vi "HandleObservationSync.vi"(8 "error in (no error)":errorcluster, 11 "S4GUI in":refnum<class "S4GUI.lvclass">) -> (0 "error out":errorcluster, 3 "S4GUI out":refnum<class "S4GUI.lvclass">)   [LabVIEW 2018, in "S4GUI.lvclass"] (continued)
              n1024 = call-dynamic "Read State Machine.vi"("error in (no error)"=w2764, "Device in"=w2765) -> ("error out"=w2763:errorcluster, "State Machine.lvclass"=w2761:refnum<class "State Machine.lvclass">, "Device out"=w2767:refnum<class "Channel.lvclass">)  [unwired: 7 in]
              n1025 = call "Next State.vi"("error in (no error)"=w2763, "New_State"=50, "State Machine in"=w2761) -> ("error out"=w2755:errorcluster, "State Machine out"=w2754:refnum<class "State Machine.lvclass">)  [unwired: 7 in]
              n1026 = call-dynamic "Write State Machine.vi"("error in (no error)"=w2755, "State Machine.lvclass"=w2754, "Device in"=w2767) -> ("error out"=w2768:errorcluster, "Device out"=w2766:refnum<class "Channel.lvclass">)  [unwired: 7 in]
              n1027 = call-dynamic "Write Channel.vi"("error in (no error)"=w2768, "Channel.lvclass"=w2766, "Acquisition in"=w2758) -> ("error out"=w2760:errorcluster, "Acquisition out"=w2759:refnum<class "Acquisition.lvclass">)  [unwired: 7 in]
            }
          }
          n1028 = call-dynamic "Write AcquisitionC.vi"("error in (no error)"=w2679, "Acquisition.lvclass"=w2677, "S4ACS_GUI in"=w2678) -> ("error out"=w2673:errorcluster, "S4ACS_GUI out"=w2672:refnum<class "S4GUI.lvclass">)  [unwired: 7 in]
          n1029 = call-dynamic "Read AcquisitionD.vi"("error in (no error)"=w2673, "S4ACS_GUI in"=w2672) -> ("error out"=w2629:errorcluster, "Acquisition.lvclass"=w2631:refnum<class "Acquisition.lvclass">, "S4ACS_GUI out"=w2671:refnum<class "S4GUI.lvclass">)  [unwired: 7 in]
          n1030 = call-dynamic "Read enabled.vi"("error in (no error)"=w2629, "Server in"=w2631) -> ("error out"=w2628:errorcluster, "enabled"=w2624:bool, "Server out"=w2630:refnum<class "Acquisition.lvclass">)  [unwired: 7 in]
          n1031 = call "Read connection.vi"("error in (no error)"=w2628, "Server in"=w2630) -> ("error out"=w2660:errorcluster, "connection"=w2644:bool, "Server out"=w2661:refnum<class "Acquisition.lvclass">)  [unwired: 7 in]
          n1032 = And(x=w2644, y=w2624) -> (x .and. y?=w2646:bool)
          n1033 = case shown="True" w2646 {
            tunnel: w2660 -> [w2729 w2746]
            tunnel: [w2729 w2745] -> w2674
            tunnel: w2661 -> [w2730 w2736]
            tunnel: [w2730 w2734] -> w2670
            tunnel: [w2726 u32 0 ("New_State")] -> w2653
            tunnel: w2624 -> [w2725 _]
            frame False {
              n1034 = Select(t=u32 8, s=w2725, f=u32 0) -> (s? t:f=w2726:u32)
            }
            frame True {
              n1035 = call-dynamic "Read Channel.vi"("error in (no error)"=w2746, "Acquisition in"=w2736) -> ("error out"=w2741:errorcluster, "Channel.lvclass"=w2740:refnum<class "Channel.lvclass">, "Acquisition out"=w2735:refnum<class "Acquisition.lvclass">)  [unwired: 7 in]
              n1036 = call-dynamic "Read State Machine.vi"("error in (no error)"=w2741, "Device in"=w2740) -> ("error out"=w2742:errorcluster, "State Machine.lvclass"=w2744:refnum<class "State Machine.lvclass">, "Device out"=w2738:refnum<class "Channel.lvclass">)  [unwired: 7 in]
              n1037 = call "Next State.vi"("error in (no error)"=w2742, "New_State"=50, "State Machine in"=w2744) -> ("error out"=w2732:errorcluster, "State Machine out"=w2733:refnum<class "State Machine.lvclass">)  [unwired: 7 in]
              n1038 = call-dynamic "Write State Machine.vi"("error in (no error)"=w2732, "State Machine.lvclass"=w2733, "Device in"=w2738) -> ("error out"=w2737:errorcluster, "Device out"=w2739:refnum<class "Channel.lvclass">)  [unwired: 7 in]
              n1039 = call-dynamic "Write Channel.vi"("error in (no error)"=w2737, "Channel.lvclass"=w2739, "Acquisition in"=w2735) -> ("error out"=w2745:errorcluster, "Acquisition out"=w2734:refnum<class "Acquisition.lvclass">)  [unwired: 7 in]
            }
          }
          n1040 = call-dynamic "Write AcquisitionD.vi"("error in (no error)"=w2674, "Acquisition.lvclass"=w2670, "S4ACS_GUI in"=w2671) -> ("error out"=w2669:errorcluster, "S4ACS_GUI out"=w2668:refnum<class "S4GUI.lvclass">)  [unwired: 7 in]
          n1041 = Compound Arithmetic op=ADD(w2656, w2655, w2654, w2653) -> (w2657:u32)
          n1042 = case shown="0, Default" w2657 {
            tunnel: w2652 -> [w2694 _ _ _ _ _ _ _ _ _ _ _ _ _ _ _]
            tunnel: [w2693 u32 1 ("Obs_state") u32 1 ("Obs_state") u32 1 ("Obs_state") u32 1 ("Obs_state") u32 1 ("Obs_state") u32 1 ("Obs_state") u32 1 ("Obs_state") u32 1 ("Obs_state") u32 1 ("Obs_state") u32 1 ("Obs_state") u32 1 ("Obs_state") u32 1 ("Obs_state") u32 1 ("Obs_state") u32 1 ("Obs_state") u32 1 ("Obs_state")] -> w2658
            tunnel: ["" ("Error Msg") "ERROR: Lost channel 1 connection... - HandleObservationSync.vi state 308" ("Error Msg") "ERROR: Lost channel 2 connection...- HandleObservationSync.vi state 308" ("Error Msg") "ERROR: Lost channels 1 and 2 connection...- HandleObservationSync.vi state 308" ("Error Msg") "ERROR: Lost channel 3 connection...- HandleObservationSync.vi state 308" ("Error Msg") "ERROR: Lost channels 1 and  3 connection...- HandleObservationSync.vi state 308" ("Error Msg") "ERROR:  Lost channels 2 and  3 connection...- HandleObservationSync.vi state 308" ("Error Msg") "ERROR:  Lost channels 1, 2 and  3 connection...- HandleObservationSync.vi state 308" ("Error Msg") "ERROR: Lost channel 4 connection...- HandleObservationSync.vi state 308" ("Error Msg") "ERROR:  Lost channels 1 and 4 connection...- HandleObservationSync.vi state 308" ("Error Msg") "ERROR:  Lost channels 2 and 4 connection...- HandleObservationSync.vi state 308" ("Error Msg") "ERROR: Lost channels 1, 2 and 4 connection...- HandleObservationSync.vi state 308" ("Error Msg") "ERROR: Lost channels 3 and 4 connection...- HandleObservationSync.vi state 308" ("Error Msg") "ERROR: Lost channels 1, 3 and 4 connection...- HandleObservationSync.vi state 308" ("Error Msg") "ERROR: Lost channels 2, 3 and 4 connection...- HandleObservationSync.vi state 308" ("Error Msg") "ERROR: Lost channels 1, 2, 3 and 4 connection...- HandleObservationSync.vi state 308" ("Error Msg")] -> w2659
            frame 0, Default {
              n1043 = Tick Count (ms)() -> (millisecond timer value=w2691:u32)
              n1044 = Increment(x=w2694) -> (x+1=w2693:u32)
              n1045 = local write "time1"(w2691) -> ()
            }
            frame 1 {
            }
            frame 2 {
            }
            frame 3 {
            }
            frame 4 {
            }
            frame 5 {
            }
            frame 6 {
            }
            frame 7 {
            }
            frame 8 {
            }
            frame 9 {
            }
            frame 10 {
            }
            frame 11 {
            }
            frame 12 {
            }
            frame 13 {
            }
            frame 14 {
            }
            frame 15 {
            }
          }
          n1046 = Bundle By Name(cluster=w2668, "Obs_state"=w2658, "Error Msg"=w2659) -> (w2685:refnum<class "S4GUI.lvclass">)
        }
        frame 309 {
          # "Se wait_expose=T, não envia\no EXPOSE do estado 310\n(1o EXPOSE já foi enviado).\n\nNeste caso, vai para:\n* 310 se houver mais \n   de 1 posição da lamina ou para \n* 327 se houver apenas 1 posição\n   da lâmina"
          # "T: mode EXPOSE\nF: mode FIRE"
          n1047 = Unbundle By Name(w2819) -> ("seqAtual"=w2818:u32)
          n1048 = call-dynamic "Read AcquisitionA.vi"("error in (no error)"=w2879, "S4ACS_GUI in"=w2819) -> ("error out"=w2859:errorcluster, "Acquisition.lvclass"=w2860:refnum<class "Acquisition.lvclass">, "S4ACS_GUI out"=w2881:refnum<class "S4GUI.lvclass">)  [unwired: 7 in]
          n1049 = call "Read connection.vi"("error in (no error)"=w2859, "Server in"=w2860) -> ("error out"=w2861:errorcluster, "connection"=w2863:bool, "Server out"=w2862:refnum<class "Acquisition.lvclass">)  [unwired: 7 in]
          n1050 = case shown="True" w2863 {
            tunnel: [w3032 w3056] -> w2882
            tunnel: [w3031 w3055] -> w2880
            tunnel: w2862 -> [w3032 w3048]
            tunnel: w2861 -> [w3031 w3047]
            tunnel: [TRUE w3046] -> w2842
            tunnel: [FALSE w3040] -> w2838
            tunnel: [TRUE w3034] -> w2823
            tunnel: w2818 -> [_ w3033]
            frame False {
            }
            frame True {
              n1051 = call-dynamic "Read Channel.vi"("error in (no error)"=w3047, "Acquisition in"=w3048) -> ("error out"=w3037:errorcluster, "Channel.lvclass"=w3039:refnum<class "Channel.lvclass">, "Acquisition out"=w3057:refnum<class "Acquisition.lvclass">)  [unwired: 7 in]
              n1052 = call-dynamic "Read SequesDone.vi"("error in (no error)"=w3037, "Channel in"=w3039) -> ("error out"=w3036:errorcluster, "SequesDoneRaw"=w3035:u32, "Channel out"=w3038:refnum<class "Channel.lvclass">)  [unwired: 6 in, 1 out]
              n1053 = Equal?(x=w3035, y=w3033) -> (x = y?=w3034:bool)
              n1054 = call-dynamic "Read wait_expose.vi"("error in (no error)"=w3036, "Channel in"=w3038) -> ("error out"=w3041:errorcluster, "wait_expose"=w3040:bool, "Channel out"=w3042:refnum<class "Channel.lvclass">)  [unwired: 7 in]
              n1055 = call-dynamic "Read State Machine.vi"("error in (no error)"=w3041, "Device in"=w3042) -> ("error out"=w3049:errorcluster, "State Machine.lvclass"=w3051:refnum<class "State Machine.lvclass">, "Device out"=w3053:refnum<class "Channel.lvclass">)  [unwired: 7 in]
              n1056 = call-dynamic "Read State.vi"("error in (no error)"=w3049, "State Machine in"=w3051) -> ("error out"=w3043:errorcluster, "State"=w3045:i32, "State Machine out"=w3050:refnum<class "State Machine.lvclass">)  [unwired: 7 in]
              n1057 = Greater?(x=w3045, y=53) -> (0:w3046:bool)
              n1058 = call-dynamic "Write State Machine.vi"("error in (no error)"=w3043, "State Machine.lvclass"=w3050, "Device in"=w3053) -> ("error out"=w3052:errorcluster, "Device out"=w3054:refnum<class "Channel.lvclass">)  [unwired: 7 in]
              n1059 = call-dynamic "Write Channel.vi"("error in (no error)"=w3052, "Channel.lvclass"=w3054, "Acquisition in"=w3057) -> ("error out"=w3055:errorcluster, "Acquisition out"=w3056:refnum<class "Acquisition.lvclass">)  [unwired: 7 in]
            }
          }
          n1060 = call-dynamic "Write AcquisitionA.vi"("error in (no error)"=w2880, "Acquisition.lvclass"=w2882, "S4ACS_GUI in"=w2881) -> ("error out"=w2876:errorcluster, "S4ACS_GUI out"=w2877:refnum<class "S4GUI.lvclass">)  [unwired: 7 in]
          n1061 = call "Read AcquisitionB.vi"("error in (no error)"=w2876, "S4ACS_GUI in"=w2877) -> ("error out"=w2856:errorcluster, "Acquisition.lvclass"=w2858:refnum<class "Acquisition.lvclass">, "S4ACS_GUI out"=w2874:refnum<class "S4GUI.lvclass">)  [unwired: 7 in]
          n1062 = call "Read connection.vi"("error in (no error)"=w2856, "Server in"=w2858) -> ("error out"=w2855:errorcluster, "connection"=w2854:bool, "Server out"=w2857:refnum<class "Acquisition.lvclass">)  [unwired: 7 in]
          n1063 = case shown="True" w2854 {
            tunnel: w2857 -> [w3002 w3027]
            tunnel: w2855 -> [w3001 w3026]
            tunnel: [w3002 w3024] -> w2875
            tunnel: [w3001 w3023] -> w2873
            tunnel: [TRUE w3014] -> w2841
            tunnel: [FALSE ("expose") w3010] -> w2837
            tunnel: [TRUE w3004] -> w2825
            tunnel: w2818 -> [_ w3003]
            frame False {
            }
            frame True {
              n1064 = call-dynamic "Read Channel.vi"("error in (no error)"=w3026, "Acquisition in"=w3027) -> ("error out"=w3006:errorcluster, "Channel.lvclass"=w3009:refnum<class "Channel.lvclass">, "Acquisition out"=w3025:refnum<class "Acquisition.lvclass">)  [unwired: 7 in]
              n1065 = call-dynamic "Read SequesDone.vi"("error in (no error)"=w3006, "Channel in"=w3009) -> ("error out"=w3005:errorcluster, "SequesDoneRaw"=w3007:u32, "Channel out"=w3008:refnum<class "Channel.lvclass">)  [unwired: 6 in, 1 out]
              n1066 = Equal?(x=w3007, y=w3003) -> (x = y?=w3004:bool)
              n1067 = call-dynamic "Read wait_expose.vi"("error in (no error)"=w3005, "Channel in"=w3008) -> ("error out"=w3011:errorcluster, "wait_expose"=w3010:bool, "Channel out"=w3012:refnum<class "Channel.lvclass">)  [unwired: 7 in]
              n1068 = call-dynamic "Read State Machine.vi"("error in (no error)"=w3011, "Device in"=w3012) -> ("error out"=w3017:errorcluster, "State Machine.lvclass"=w3019:refnum<class "State Machine.lvclass">, "Device out"=w3021:refnum<class "Channel.lvclass">)  [unwired: 7 in]
              n1069 = call-dynamic "Read State.vi"("error in (no error)"=w3017, "State Machine in"=w3019) -> ("error out"=w3016:errorcluster, "State"=w3013:i32, "State Machine out"=w3018:refnum<class "State Machine.lvclass">)  [unwired: 7 in]
              n1070 = Greater?(x=w3013, y=53) -> (0:w3014:bool)
              n1071 = call-dynamic "Write State Machine.vi"("error in (no error)"=w3016, "State Machine.lvclass"=w3018, "Device in"=w3021) -> ("error out"=w3020:errorcluster, "Device out"=w3022:refnum<class "Channel.lvclass">)  [unwired: 7 in]
              n1072 = call-dynamic "Write Channel.vi"("error in (no error)"=w3020, "Channel.lvclass"=w3022, "Acquisition in"=w3025) -> ("error out"=w3023:errorcluster, "Acquisition out"=w3024:refnum<class "Acquisition.lvclass">)  [unwired: 7 in]
            }
          }
          n1073 = call "Write AcquisitionB.vi"("error in (no error)"=w2873, "Acquisition.lvclass"=w2875, "S4ACS_GUI in"=w2874) -> ("error out"=w2869:errorcluster, "S4ACS_GUI out"=w2868:refnum<class "S4GUI.lvclass">)  [unwired: 7 in]
          n1074 = call-dynamic "Read AcquisitionC.vi"("error in (no error)"=w2869, "S4ACS_GUI in"=w2868) -> ("error out"=w2851:errorcluster, "Acquisition.lvclass"=w2853:refnum<class "Acquisition.lvclass">, "S4ACS_GUI out"=w2871:refnum<class "S4GUI.lvclass">)  [unwired: 7 in]
          n1075 = call "Read connection.vi"("error in (no error)"=w2851, "Server in"=w2853) -> ("error out"=w2850:errorcluster, "connection"=w2849:bool, "Server out"=w2852:refnum<class "Acquisition.lvclass">)  [unwired: 7 in]
          n1076 = case shown="True" w2849 {
            tunnel: [w2971 w2992] -> w2872
            tunnel: [w2972 w2991] -> w2870
            tunnel: w2852 -> [w2972 w2987]
            tunnel: w2850 -> [w2971 w2986]
            tunnel: [TRUE w2983] -> w2840
            tunnel: [FALSE ("expose") w2980] -> w2836
            tunnel: [TRUE w2974] -> w2824
            tunnel: w2818 -> [_ w2973]
            frame False {
            }
            frame True {
              n1077 = call-dynamic "Read Channel.vi"("error in (no error)"=w2986, "Acquisition in"=w2987) -> ("error out"=w2979:errorcluster, "Channel.lvclass"=w2978:refnum<class "Channel.lvclass">, "Acquisition out"=w2990:refnum<class "Acquisition.lvclass">)  [unwired: 7 in]
              n1078 = call-dynamic "Read SequesDone.vi"("error in (no error)"=w2979, "Channel in"=w2978) -> ("error out"=w2975:errorcluster, "SequesDoneRaw"=w2976:u32, "Channel out"=w2977:refnum<class "Channel.lvclass">)  [unwired: 6 in, 1 out]
              n1079 = Equal?(x=w2976, y=w2973) -> (x = y?=w2974:bool)
              n1080 = call-dynamic "Read wait_expose.vi"("error in (no error)"=w2975, "Channel in"=w2977) -> ("error out"=w2981:errorcluster, "wait_expose"=w2980:bool, "Channel out"=w2982:refnum<class "Channel.lvclass">)  [unwired: 7 in]
              n1081 = call-dynamic "Read State Machine.vi"("error in (no error)"=w2981, "Device in"=w2982) -> ("error out"=w2988:errorcluster, "State Machine.lvclass"=w2996:refnum<class "State Machine.lvclass">, "Device out"=w2994:refnum<class "Channel.lvclass">)  [unwired: 7 in]
              n1082 = call-dynamic "Read State.vi"("error in (no error)"=w2988, "State Machine in"=w2996) -> ("error out"=w2989:errorcluster, "State"=w2984:i32, "State Machine out"=w2997:refnum<class "State Machine.lvclass">)  [unwired: 7 in]
              n1083 = Greater?(x=w2984, y=53) -> (0:w2983:bool)
              n1084 = call-dynamic "Write State Machine.vi"("error in (no error)"=w2989, "State Machine.lvclass"=w2997, "Device in"=w2994) -> ("error out"=w2995:errorcluster, "Device out"=w2993:refnum<class "Channel.lvclass">)  [unwired: 7 in]
              n1085 = call-dynamic "Write Channel.vi"("error in (no error)"=w2995, "Channel.lvclass"=w2993, "Acquisition in"=w2990) -> ("error out"=w2992:errorcluster, "Acquisition out"=w2991:refnum<class "Acquisition.lvclass">)  [unwired: 7 in]
            }
          }
          n1086 = call-dynamic "Write AcquisitionC.vi"("error in (no error)"=w2872, "Acquisition.lvclass"=w2870, "S4ACS_GUI in"=w2871) -> ("error out"=w2848:errorcluster, "S4ACS_GUI out"=w2864:refnum<class "S4GUI.lvclass">)  [unwired: 7 in]
          n1087 = call-dynamic "Read AcquisitionD.vi"("error in (no error)"=w2848, "S4ACS_GUI in"=w2864) -> ("error out"=w2844:errorcluster, "Acquisition.lvclass"=w2847:refnum<class "Acquisition.lvclass">, "S4ACS_GUI out"=w2866:refnum<class "S4GUI.lvclass">)  [unwired: 7 in]
          n1088 = call "Read connection.vi"("error in (no error)"=w2844, "Server in"=w2847) -> ("error out"=w2845:errorcluster, "connection"=w2843:bool, "Server out"=w2846:refnum<class "Acquisition.lvclass">)  [unwired: 7 in]
          n1089 = case shown="True" w2843 {
            tunnel: [w2942 w2966] -> w2867
            tunnel: [w2941 w2965] -> w2865
            tunnel: [TRUE w2954] -> w2839
            tunnel: w2846 -> [w2942 w2957]
            tunnel: w2845 -> [w2941 w2956]
            tunnel: [FALSE ("expose") w2950] -> w2835
            tunnel: [TRUE w2944] -> w2826
            tunnel: w2818 -> [_ w2943]
            frame False {
            }
            frame True {
              n1090 = call-dynamic "Read Channel.vi"("error in (no error)"=w2956, "Acquisition in"=w2957) -> ("error out"=w2948:errorcluster, "Channel.lvclass"=w2949:refnum<class "Channel.lvclass">, "Acquisition out"=w2967:refnum<class "Acquisition.lvclass">)  [unwired: 7 in]
              n1091 = call-dynamic "Read SequesDone.vi"("error in (no error)"=w2948, "Channel in"=w2949) -> ("error out"=w2946:errorcluster, "SequesDoneRaw"=w2947:u32, "Channel out"=w2945:refnum<class "Channel.lvclass">)  [unwired: 6 in, 1 out]
              n1092 = Equal?(x=w2947, y=w2943) -> (x = y?=w2944:bool)
              n1093 = call-dynamic "Read wait_expose.vi"("error in (no error)"=w2946, "Channel in"=w2945) -> ("error out"=w2951:errorcluster, "wait_expose"=w2950:bool, "Channel out"=w2952:refnum<class "Channel.lvclass">)  [unwired: 7 in]
              n1094 = call-dynamic "Read State Machine.vi"("error in (no error)"=w2951, "Device in"=w2952) -> ("error out"=w2959:errorcluster, "State Machine.lvclass"=w2961:refnum<class "State Machine.lvclass">, "Device out"=w2963:refnum<class "Channel.lvclass">)  [unwired: 7 in]
              n1095 = call-dynamic "Read State.vi"("error in (no error)"=w2959, "State Machine in"=w2961) -> ("error out"=w2958:errorcluster, "State"=w2953:i32, "State Machine out"=w2960:refnum<class "State Machine.lvclass">)  [unwired: 7 in]
              n1096 = Greater?(x=w2953, y=53) -> (0:w2954:bool)
              n1097 = call-dynamic "Write State Machine.vi"("error in (no error)"=w2958, "State Machine.lvclass"=w2960, "Device in"=w2963) -> ("error out"=w2962:errorcluster, "Device out"=w2964:refnum<class "Channel.lvclass">)  [unwired: 7 in]
              n1098 = call-dynamic "Write Channel.vi"("error in (no error)"=w2962, "Channel.lvclass"=w2964, "Acquisition in"=w2967) -> ("error out"=w2965:errorcluster, "Acquisition out"=w2966:refnum<class "Acquisition.lvclass">)  [unwired: 7 in]
            }
          }
          n1099 = call-dynamic "Write AcquisitionD.vi"("error in (no error)"=w2865, "Acquisition.lvclass"=w2867, "S4ACS_GUI in"=w2866) -> ("error out"=w2817:errorcluster, "S4ACS_GUI out"=w2815:refnum<class "S4GUI.lvclass">)  [unwired: 7 in]
          n1100 = Compound Arithmetic op=OR(w2838, w2837, w2836, w2835) -> (w2828:bool)
          n1101 = Compound Arithmetic op=AND(w2823, w2825, w2824, w2826) -> (w2821:bool)
          n1102 = Compound Arithmetic op=AND(w2842, w2841, w2840, w2839) -> (w2822:bool)
          n1103 = disable-structure shown="Enabled" {
            disable-tunnel: w2822 -> [w2885 w2886]
            disable-tunnel: w2821 -> [w2884 _]
            disable-tunnel: [w2883 w2886] -> w2820
            frame Disabled {
              # "Espera todos os canais chegarem ao estado ACTIVE\n(estados 54 e 55 de Channel:Run.vi)\n   OU\nTodos os canais incrementarem o Seqs_done. (OV 20240821)"
              n1104 = Or(x=w2885, y=w2884) -> (x .or. y?=w2883:bool)
            }
            frame Enabled {
              # "OV20241108:\nEspera APENAS o ACTIVE."
            }
          }
          n1105 = call-dynamic "VerifErrors.vi"("error in (no error)"=w2817, "S4GUI in"=w2815) -> ("error out"=w2816:errorcluster, "Error value"=w2813:u32, "S4GUI out"=w2814:refnum<class "S4GUI.lvclass">)  [unwired: 7 in]
          n1106 = call-dynamic "VerifWavePlate.vi"("error in (no error)"=w2816, "S4GUI in"=w2814) -> ("error out"=w2832:errorcluster, "One Position"=w2834:bool, "S4GUI out"=w2833:refnum<class "S4GUI.lvclass">)  [unwired: 7 in]
          n1107 = case shown="False" w2834 {
            tunnel: w2833 -> [w2919 w2936]
            tunnel: [u32 312 ("t") u32 328 ("t")] -> w2830
            tunnel: [w2919 w2922] -> w2829
            tunnel: w2832 -> [w2917 w2921]
            tunnel: [w2917 w2920] -> w2831
            frame False {
            }
            frame True {
              # "Recarrega SEQ, antes de desviar\n para tratamento de fotometria."
              n1108 = call "Read Instrument.lvclass.vi"("error in (no error)"=w2921, "S4ACS_GUI in"=w2936) -> ("error out"=w2931:errorcluster, "Instrument.lvclass"=w2935:refnum<class "Instrument.lvclass">, "S4ACS_GUI out"=w2934:refnum<class "S4GUI.lvclass">)  [unwired: 7 in]
              n1109 = call "Read WPROT.vi"("error in (no error)"=w2931, "Instrument in"=w2935) -> ("error out"=w2924:errorcluster, "Opt_Selector.lvclass"=w2927:refnum<class "Opt_Selector.lvclass">, "Instrument out"=w2932:refnum<class "Instrument.lvclass">)  [unwired: 7 in]
              n1110 = call-dynamic "Read sequencia_ant.vi"("error in (no error)"=w2924, "Opt_Selector in"=w2927) -> ("error out"=w2929:errorcluster, "sequencia_ant"=w2928:u16, "Opt_Selector out"=w2926:refnum<class "Opt_Selector.lvclass">)  [unwired: 7 in]
              n1111 = call-dynamic "Write sequencia.vi"("error in (no error)"=w2929, "sequencia"=w2928, "Opt_Selector in"=w2926) -> ("error out"=w2923:errorcluster, "Opt_Selector out"=w2925:refnum<class "Opt_Selector.lvclass">)  [unwired: 7 in]
              n1112 = call "Write WPROT.vi"("error in (no error)"=w2923, "Opt_Selector.lvclass"=w2925, "Instrument in"=w2932) -> ("error out"=w2930:errorcluster, "Instrument out"=w2933:refnum<class "Instrument.lvclass">)  [unwired: 7 in]
              n1113 = call "Write Instrument.lvclass.vi"("error in (no error)"=w2930, "Instrument.lvclass"=w2933, "S4ACS_GUI in"=w2934) -> ("error out"=w2920:errorcluster, "S4ACS_GUI out"=w2922:refnum<class "S4GUI.lvclass">)  [unwired: 7 in]
            }
          }
          n1114 = case shown="False" w2820 {
            tunnel: w2829 -> [w2889 w2916]
            tunnel: [w2895 w2915] -> w2827
            tunnel: w2830 -> [_ w2913]
            tunnel: w2813 -> [w2887 _]
            frame False {
              # "Aguardando iniciar exposição por 5s"
              n1115 = Tick Count (ms)() -> (millisecond timer value=w2894:u32)
              n1116 = local read "time1"() -> (w2888:u32)
              n1117 = Subtract(x=w2894, y=w2888) -> (x-y=w2891:u32)
              n1118 = To Double Precision Float(number=w2891) -> (double precision float=w2893:dbl)
              n1119 = Less?(x=5000.0 ("y"), y=w2893) -> (x < y?=w2892:bool)
              n1120 = case shown="False" w2892 {
                tunnel: w2889 -> [w2897 w2911]
                tunnel: [w2896 w2910] -> w2895
                tunnel: w2887 -> [w2898 _]
                frame False {
                  n1121 = case shown="1..15" w2898 {
                    selector: w2898 -> [_ w2906]
                    tunnel: [w2899 w2901] -> w2896
                    tunnel: w2897 -> [w2899 w2907]
                    frame 0, Default {
                    }
                    frame 1..15 {
                      n1122 = Number To Decimal String(number=w2906) -> (decimal integer string=w2903:string)  [unwired: 1 in]
                      n1123 = Concatenate Strings("CHANNEL ERROR <", w2903, ">: Error flag TRUE - see ACS panel.  HandleObservationSync.vi - state 309.") -> (w2905:string)
                      n1124 = Bundle By Name(cluster=w2907, "Obs_state"=u32 1, "Error Msg"=w2905) -> (w2901:refnum<class "S4GUI.lvclass">)
                    }
                  }
                }
                frame True {
                  n1125 = Bundle By Name(cluster=w2911, "Obs_state"=u32 1, "Error Msg"="ERROR: Acquisition Timeout. HandleObservationSync.vi - state 309.") -> (w2910:refnum<class "S4GUI.lvclass">)
                }
              }
            }
            frame True {
              # "Iniciou aquisição..."
              n1126 = Tick Count (ms)() -> (millisecond timer value=→"time308":u32)
              n1127 = Tick Count (ms)() -> (millisecond timer value=w2914:u32)
              n1128 = Bundle By Name(cluster=w2916, "Obs_state"=w2913) -> (w2915:refnum<class "S4GUI.lvclass">)
              n1129 = local write "time307"(w2914) -> ()
              n1130 = local write "time1"(w2914) -> ()
            }
          }
          n1131 = Bundle By Name(cluster=w2827, "mode EXPOSE"=w2828) -> (w2878:refnum<class "S4GUI.lvclass">)
        }
        frame 312 {
          # "Verifcando avanço de SEQUENCIA:"
          # "T=canais receberam STOP"
          # "T= Todos os canais ativos na mesma sequencia;\nF= Canais com sequencia diferente"
          # "Todos os SEQ_DONE \nsão iguais a SeqAtual?\nSe sim, avança lâmina."
          # "Exemplo:\nSET #CYCLES 3\nSET #SEQ 4\ntotal de sequencias: 3 x 4 = 12\n\nseq.        CYCLES_DONE           SEQS_DONE\n1a.                     0                                 0\n2a.                     0                                 1 \n3a.                     0                                 2 \n4a.                     0                                 3 \n                          1                                 4\n5a.                     1                                 0 \n6a.                     1                                 1 \n7a.                     1                                 2 \n8a.                     1                                 3 \n                          2                                 4\n9a.                     2                                 0 \n10a.                   2                                 1 \n11a.                   2                                 2 \n12a.                   2                                 3 \n\nfim                    3                                 4"
          n1132 = Unbundle By Name(w3083) -> ("seqAtual"=w3080:u32)
          n1133 = call-dynamic "Read AcquisitionA.vi"("error in (no error)"=w3117, "S4ACS_GUI in"=w3083) -> ("error out"=w3098:errorcluster, "Acquisition.lvclass"=w3099:refnum<class "Acquisition.lvclass">, "S4ACS_GUI out"=w3119:refnum<class "S4GUI.lvclass">)  [unwired: 7 in]
          n1134 = call-dynamic "Read enabled.vi"("error in (no error)"=w3098, "Server in"=w3099) -> ("error out"=w3097:errorcluster, "enabled"=w3072:bool, "Server out"=w3096:refnum<class "Acquisition.lvclass">)  [unwired: 7 in]
          n1135 = case shown="True" w3072 {
            tunnel: w3097 -> [w3268 w3284]
            tunnel: [w3269 w3282] -> w3120
            tunnel: [w3268 w3281] -> w3118
            tunnel: [u32 0 ("SequesDone") w3270] -> w3077
            tunnel: w3096 -> [w3269 w3280]
            tunnel: w3080 -> [_ w3279]
            tunnel: [TRUE w3278] -> w3082
            tunnel: [FALSE ("stopping") w3271] -> w3065
            frame False {
            }
            frame True {
              # "SEQS_DONE = 0,1,2,...,n,0,1,..."
              n1136 = call-dynamic "Read Channel.vi"("error in (no error)"=w3284, "Acquisition in"=w3280) -> ("error out"=w3276:errorcluster, "Channel.lvclass"=w3277:refnum<class "Channel.lvclass">, "Acquisition out"=w3283:refnum<class "Acquisition.lvclass">)  [unwired: 7 in]
              n1137 = call-dynamic "Read SequesDone.vi"("error in (no error)"=w3276, "Channel in"=w3277) -> ("error out"=w3274:errorcluster, "SequesDoneRaw"=w3270:u32, "Channel out"=w3275:refnum<class "Channel.lvclass">)  [unwired: 6 in, 1 out]
              n1138 = Equal?(x=w3270, y=w3279) -> (x = y?=w3278:bool)
              n1139 = call-dynamic "Read stopping.vi"("error in (no error)"=w3274, "Channel in"=w3275) -> ("error out"=w3273:errorcluster, "stopping"=w3271:bool, "Channel out"=w3272:refnum<class "Channel.lvclass">)  [unwired: 7 in]
              n1140 = call-dynamic "Write Channel.vi"("error in (no error)"=w3273, "Channel.lvclass"=w3272, "Acquisition in"=w3283) -> ("error out"=w3281:errorcluster, "Acquisition out"=w3282:refnum<class "Acquisition.lvclass">)  [unwired: 7 in]
            }
          }
          n1141 = call-dynamic "Write AcquisitionA.vi"("error in (no error)"=w3118, "Acquisition.lvclass"=w3120, "S4ACS_GUI in"=w3119) -> ("error out"=w3115:errorcluster, "S4ACS_GUI out"=w3114:refnum<class "S4GUI.lvclass">)  [unwired: 7 in]
          n1142 = call "Read AcquisitionB.vi"("error in (no error)"=w3115, "S4ACS_GUI in"=w3114) -> ("error out"=w3092:errorcluster, "Acquisition.lvclass"=w3095:refnum<class "Acquisition.lvclass">, "S4ACS_GUI out"=w3116:refnum<class "S4GUI.lvclass">)  [unwired: 7 in]
          n1143 = call-dynamic "Read enabled.vi"("error in (no error)"=w3092, "Server in"=w3095) -> ("error out"=w3093:errorcluster, "enabled"=w3071:bool, "Server out"=w3094:refnum<class "Acquisition.lvclass">)  [unwired: 7 in]
          n1144 = case shown="True" w3071 {
            tunnel: w3093 -> [w3248 w3264]
            tunnel: w3094 -> [w3249 w3263]
            tunnel: [u32 0 ("SequesDone") w3250] -> w3074
            tunnel: [w3248 w3262] -> w3113
            tunnel: [w3249 w3261] -> w3112
            tunnel: w3080 -> [_ w3258]
            tunnel: [TRUE w3257] -> w3081
            tunnel: [FALSE ("stopping") w3251] -> w3064
            frame False {
            }
            frame True {
              n1145 = call-dynamic "Read Channel.vi"("error in (no error)"=w3264, "Acquisition in"=w3263) -> ("error out"=w3255:errorcluster, "Channel.lvclass"=w3256:refnum<class "Channel.lvclass">, "Acquisition out"=w3259:refnum<class "Acquisition.lvclass">)  [unwired: 7 in]
              n1146 = call-dynamic "Read SequesDone.vi"("error in (no error)"=w3255, "Channel in"=w3256) -> ("error out"=w3253:errorcluster, "SequesDoneRaw"=w3250:u32, "Channel out"=w3260:refnum<class "Channel.lvclass">)  [unwired: 6 in, 1 out]
              n1147 = Equal?(x=w3250, y=w3258) -> (x = y?=w3257:bool)
              n1148 = call-dynamic "Read stopping.vi"("error in (no error)"=w3253, "Channel in"=w3260) -> ("error out"=w3252:errorcluster, "stopping"=w3251:bool, "Channel out"=w3254:refnum<class "Channel.lvclass">)  [unwired: 7 in]
              n1149 = call-dynamic "Write Channel.vi"("error in (no error)"=w3252, "Channel.lvclass"=w3254, "Acquisition in"=w3259) -> ("error out"=w3262:errorcluster, "Acquisition out"=w3261:refnum<class "Acquisition.lvclass">)  [unwired: 7 in]
            }
          }
          n1150 = call "Write AcquisitionB.vi"("error in (no error)"=w3113, "Acquisition.lvclass"=w3112, "S4ACS_GUI in"=w3116) -> ("error out"=w3105:errorcluster, "S4ACS_GUI out"=w3104:refnum<class "S4GUI.lvclass">)  [unwired: 7 in]
          n1151 = call-dynamic "Read AcquisitionC.vi"("error in (no error)"=w3105, "S4ACS_GUI in"=w3104) -> ("error out"=w3089:errorcluster, "Acquisition.lvclass"=w3091:refnum<class "Acquisition.lvclass">, "S4ACS_GUI out"=w3107:refnum<class "S4GUI.lvclass">)  [unwired: 7 in]
          n1152 = call-dynamic "Read enabled.vi"("error in (no error)"=w3089, "Server in"=w3091) -> ("error out"=w3088:errorcluster, "enabled"=w3070:bool, "Server out"=w3090:refnum<class "Acquisition.lvclass">)  [unwired: 7 in]
          n1153 = case shown="True" w3070 {
            tunnel: [w3228 w3244] -> w3108
            tunnel: [w3229 w3243] -> w3106
            tunnel: w3088 -> [w3228 w3240]
            tunnel: w3090 -> [w3229 w3241]
            tunnel: [u32 0 ("SequesDone") w3230] -> w3073
            tunnel: w3080 -> [_ w3239]
            tunnel: [TRUE w3238] -> w3079
            tunnel: [FALSE ("stopping") w3231] -> w3063
            frame False {
            }
            frame True {
              n1154 = call-dynamic "Read Channel.vi"("error in (no error)"=w3240, "Acquisition in"=w3241) -> ("error out"=w3235:errorcluster, "Channel.lvclass"=w3236:refnum<class "Channel.lvclass">, "Acquisition out"=w3242:refnum<class "Acquisition.lvclass">)  [unwired: 7 in]
              n1155 = call-dynamic "Read SequesDone.vi"("error in (no error)"=w3235, "Channel in"=w3236) -> ("error out"=w3233:errorcluster, "SequesDoneRaw"=w3230:u32, "Channel out"=w3237:refnum<class "Channel.lvclass">)  [unwired: 6 in, 1 out]
              n1156 = Equal?(x=w3230, y=w3239) -> (x = y?=w3238:bool)
              n1157 = call-dynamic "Read stopping.vi"("error in (no error)"=w3233, "Channel in"=w3237) -> ("error out"=w3232:errorcluster, "stopping"=w3231:bool, "Channel out"=w3234:refnum<class "Channel.lvclass">)  [unwired: 7 in]
              n1158 = call-dynamic "Write Channel.vi"("error in (no error)"=w3232, "Channel.lvclass"=w3234, "Acquisition in"=w3242) -> ("error out"=w3244:errorcluster, "Acquisition out"=w3243:refnum<class "Acquisition.lvclass">)  [unwired: 7 in]
            }
          }
          n1159 = call-dynamic "Write AcquisitionC.vi"("error in (no error)"=w3108, "Acquisition.lvclass"=w3106, "S4ACS_GUI in"=w3107) -> ("error out"=w3102:errorcluster, "S4ACS_GUI out"=w3103:refnum<class "S4GUI.lvclass">)  [unwired: 7 in]
          n1160 = call-dynamic "Read AcquisitionD.vi"("error in (no error)"=w3102, "S4ACS_GUI in"=w3103) -> ("error out"=w3085:errorcluster, "Acquisition.lvclass"=w3087:refnum<class "Acquisition.lvclass">, "S4ACS_GUI out"=w3109:refnum<class "S4GUI.lvclass">)  [unwired: 7 in]
          n1161 = call-dynamic "Read enabled.vi"("error in (no error)"=w3085, "Server in"=w3087) -> ("error out"=w3084:errorcluster, "enabled"=w3069:bool, "Server out"=w3086:refnum<class "Acquisition.lvclass">)  [unwired: 7 in]
          n1162 = Build Array(w3072, w3071, w3070, w3069) -> (w3068:bool[])
          n1163 = case shown="True" w3069 {
            tunnel: [w3209 w3224] -> w3111
            tunnel: [w3208 w3223] -> w3110
            tunnel: w3086 -> [w3209 w3222]
            tunnel: w3084 -> [w3208 w3221]
            tunnel: [u32 0 ("SequesDone") w3210] -> w3076
            tunnel: w3080 -> [_ w3219]
            tunnel: [TRUE w3218] -> w3078
            tunnel: [FALSE ("stopping") w3211] -> w3062
            frame False {
            }
            frame True {
              n1164 = call-dynamic "Read Channel.vi"("error in (no error)"=w3221, "Acquisition in"=w3222) -> ("error out"=w3215:errorcluster, "Channel.lvclass"=w3216:refnum<class "Channel.lvclass">, "Acquisition out"=w3220:refnum<class "Acquisition.lvclass">)  [unwired: 7 in]
              n1165 = call-dynamic "Read SequesDone.vi"("error in (no error)"=w3215, "Channel in"=w3216) -> ("error out"=w3213:errorcluster, "SequesDoneRaw"=w3210:u32, "Channel out"=w3217:refnum<class "Channel.lvclass">)  [unwired: 6 in, 1 out]
              n1166 = Equal?(x=w3210, y=w3219) -> (x = y?=w3218:bool)
              n1167 = call-dynamic "Read stopping.vi"("error in (no error)"=w3213, "Channel in"=w3217) -> ("error out"=w3212:errorcluster, "stopping"=w3211:bool, "Channel out"=w3214:refnum<class "Channel.lvclass">)  [unwired: 7 in]
              n1168 = call-dynamic "Write Channel.vi"("error in (no error)"=w3212, "Channel.lvclass"=w3214, "Acquisition in"=w3220) -> ("error out"=w3223:errorcluster, "Acquisition out"=w3224:refnum<class "Acquisition.lvclass">)  [unwired: 7 in]
            }
          }
          n1169 = Boolean Array To Number(Boolean array=w3068) -> (number=w3066:u32)
          n1170 = Compound Arithmetic op=AND(w3082, w3081, w3079, w3078) -> (w3067:bool)
          n1171 = Compound Arithmetic op=OR(w3065, w3064, w3063, w3062) -> (w3061:bool)
          n1172 = case shown="11" w3066 {
            tunnel: w3077 -> [w3128 _ w3140 _ w3149 _ w3155 w3161 _ w3167 w3170 _]
            tunnel: w3076 -> [w3127 w3131 w3136 w3143 w3144 w3152 w3154 _ _ _ _ _]
            tunnel: w3074 -> [w3126 w3129 _ _ w3148 w3150 _ w3160 w3164 _ w3169 _]
            tunnel: w3073 -> [w3125 w3130 w3135 w3141 _ _ _ w3159 w3163 w3166 _ _]
            tunnel: [w3121 w3132 w3137 w3142 w3145 w3151 w3153 w3156 w3162 w3165 w3168 TRUE] -> _
            frame 15 {
              # "A,B,C,D ativos"
              n1173 = Equal?(x=w3128, y=w3126) -> (x = y?=w3124:bool)
              n1174 = Equal?(x=w3125, y=w3127) -> (x = y?=w3122:bool)
              n1175 = Equal?(x=w3126, y=w3125) -> (x = y?=w3123:bool)
              n1176 = Compound Arithmetic op=AND(w3124, w3123, w3122) -> (w3121:bool)
            }
            frame 14 {
              # "B,C e,D ativos"
              n1177 = Equal?(x=w3129, y=w3130) -> (x = y?=w3134:bool)
              n1178 = Equal?(x=w3130, y=w3131) -> (x = y?=w3133:bool)
              n1179 = Compound Arithmetic op=AND(w3134, w3133) -> (w3132:bool)
            }
            frame 13 {
              # "A,C e,D ativos"
              n1180 = Equal?(x=w3140, y=w3135) -> (x = y?=w3139:bool)
              n1181 = Equal?(x=w3135, y=w3136) -> (x = y?=w3138:bool)
              n1182 = Compound Arithmetic op=AND(w3139, w3138) -> (w3137:bool)
            }
            frame 12 {
              # "Só C e D ativos"
              n1183 = Equal?(x=w3141, y=w3143) -> (x = y?=w3142:bool)
            }
            frame 11 {
              # "A,B e,D ativos"
              n1184 = Equal?(x=w3149, y=w3148) -> (x = y?=w3147:bool)
              n1185 = Equal?(x=w3148, y=w3144) -> (x = y?=w3146:bool)
              n1186 = Compound Arithmetic op=AND(w3147, w3146) -> (w3145:bool)
            }
            frame 10 {
              # "Só B e D ativos"
              n1187 = Equal?(x=w3150, y=w3152) -> (x = y?=w3151:bool)
            }
            frame 9 {
              # "Só A e D ativos"
              n1188 = Equal?(x=w3155, y=w3154) -> (x = y?=w3153:bool)
            }
            frame 7 {
              # "A,B,C ativos"
              n1189 = Equal?(x=w3161, y=w3160) -> (x = y?=w3158:bool)
              n1190 = Equal?(x=w3160, y=w3159) -> (x = y?=w3157:bool)
              n1191 = Compound Arithmetic op=AND(w3158, w3157) -> (w3156:bool)
            }
            frame 6 {
              # "Só B e C ativos"
              n1192 = Equal?(x=w3164, y=w3163) -> (x = y?=w3162:bool)
            }
            frame 5 {
              # "Só A e C ativos"
              n1193 = Equal?(x=w3167, y=w3166) -> (x = y?=w3165:bool)
            }
            frame 3 {
              # "só A e B ativos"
              n1194 = Equal?(x=w3170, y=w3169) -> (x = y?=w3168:bool)
            }
            frame 0..2, 4, 8, Default {
              # "nenhum ou só 1  \ncanal ativo."
            }
          }
          n1195 = call-dynamic "Write AcquisitionD.vi"("error in (no error)"=w3110, "Acquisition.lvclass"=w3111, "S4ACS_GUI in"=w3109) -> ("error out"=w3100:errorcluster, "S4ACS_GUI out"=w3101:refnum<class "S4GUI.lvclass">)  [unwired: 7 in]
          n1196 = And(x=w3067, y=TRUE) -> (x .and. y?=w3075:bool)
          n1197 = case shown="True" w3075 {
            tunnel: w3101 -> [w3173 w3202]
            tunnel: [w3172 w3201] -> w3060
            tunnel: w3067 -> [w3174 _]
            tunnel: w3061 -> [_ w3200]
            tunnel: w3059 -> [_ w3195]
            frame False {
              n1198 = case shown="True" w3174 {
                tunnel: w3173 -> [w3181 w3194]
                tunnel: [w3185 w3193] -> w3172
                frame False {
                  # "Esperando todos os canais habilitados mudarem de sequesDone.\nE verificando a maior duracao de cubo entre os canais."
                  n1199 = local read "time307"() -> (w3184:u32)
                  n1200 = Tick Count (ms)() -> (millisecond timer value=w3183:u32)
                  n1201 = Subtract(x=w3183, y=w3184) -> (x-y=w3178:u32)
                  n1202 = call-dynamic "GetGreatestCube.vi"("S4GUI in"=w3181) -> ("S4GUI out"=w3180:refnum<class "S4GUI.lvclass">, "greatest (ms)"=w3176:dbl)  [unwired: 8 in, 1 out]
                  n1203 = To Double Precision Float(number=w3178) -> (double precision float=w3182:dbl)
                  n1204 = Add(x=1000.0 ("y"), y=w3176) -> (x+y=w3175:dbl)
                  n1205 = Less?(x=w3175, y=w3182) -> (x < y?=w3179:bool)
                  n1206 = case shown="True" w3179 {
                    tunnel: w3180 -> [w3186 w3190]
                    tunnel: [w3186 w3189] -> w3185
                    frame False {
                    }
                    frame True {
                      n1207 = Bundle By Name(cluster=w3190, "Obs_state"=u32 1, "Error Msg"="ERROR: Acquisition Timeout - HandleObservationSync.vi - state 312.") -> (w3189:refnum<class "S4GUI.lvclass">)
                    }
                  }
                }
                frame True {
                  # "Nunca entra aqui!!"
                  n1208 = Bundle By Name(cluster=w3194, "Obs_state"=u32 1, "Error Msg"="ERROR: Sequence_done not equal in all active channels.") -> (w3193:refnum<class "S4GUI.lvclass">)
                }
              }
            }
            frame True {
              # "STOP?"
              n1209 = local read "time308"() -> (w3198:u32)
              n1210 = Tick Count (ms)() -> (millisecond timer value=w3199:u32)
              n1211 = Subtract(x=w3199, y=w3198) -> (x-y=→"delay Acq":u32)
              n1212 = case shown="False" w3200 {
                tunnel: w3195 -> [_ _]
                tunnel: [u32 303 u32 0] -> w3196
                frame False {
                }
                frame True {
                }
              }
              n1213 = Bundle By Name(cluster=w3202, "Obs_state"=w3196) -> (w3201:refnum<class "S4GUI.lvclass">)
            }
          }
        }
        frame 314 {
          n1214 = Unbundle By Name(w3288) -> ("cyclesDone"=w3286:u32)
          n1215 = Increment(x=w3286) -> (x+1=w3285:u32)
          n1216 = Bundle By Name(cluster=w3288, "cyclesDone"=w3285) -> (w3287:refnum<class "S4GUI.lvclass">)
          n1217 = Unbundle By Name(w3287) -> ("TotalCiclos"=w3295:u32, "cyclesDone"=w3294:u32)
          n1218 = Subtract(x=w3295, y=w3294) -> (x-y=w3293:u32)
          n1219 = Greater Than 0?(x=w3293) -> (x > 0?=w3292:bool)
          n1220 = Select(t=u32 303, s=w3292, f=u32 0) -> (s? t:f=w3291:u32)
          n1221 = Bundle By Name(cluster=w3287, "Obs_state"=w3291) -> (w3296:refnum<class "S4GUI.lvclass">)
        }
        frame 321 {
          n1222 = call-dynamic "Read AcquisitionA.vi"("error in (no error)"=w3360, "S4ACS_GUI in"=w3361) -> ("error out"=w3315:errorcluster, "Acquisition.lvclass"=w3316:refnum<class "Acquisition.lvclass">, "S4ACS_GUI out"=w3363:refnum<class "S4GUI.lvclass">)  [unwired: 7 in]
          n1223 = call-dynamic "Read enabled.vi"("error in (no error)"=w3315, "Server in"=w3316) -> ("error out"=w3314:errorcluster, "enabled"=w3301:bool, "Server out"=w3317:refnum<class "Acquisition.lvclass">)  [unwired: 7 in]
          n1224 = call "Read connection.vi"("error in (no error)"=w3314, "Server in"=w3317) -> ("error out"=w3340:errorcluster, "connection"=w3324:bool, "Server out"=w3341:refnum<class "Acquisition.lvclass">)  [unwired: 7 in]
          n1225 = And(x=w3324, y=w3301) -> (x .and. y?=w3325:bool)
          n1226 = case shown="True" w3325 {
            tunnel: w3341 -> [w3478 w3497]
            tunnel: w3340 -> [w3477 w3496]
            tunnel: [w3478 w3494] -> w3364
            tunnel: [w3477 w3493] -> w3362
            tunnel: [w3474 u32 0 ("New_State")] -> w3330
            tunnel: w3301 -> [w3473 _]
            frame False {
              n1227 = Select(t=u32 1, s=w3473, f=u32 0) -> (s? t:f=w3474:u32)
            }
            frame True {
              n1228 = call-dynamic "Read Channel.vi"("error in (no error)"=w3496, "Acquisition in"=w3497) -> ("error out"=w3480:errorcluster, "Channel.lvclass"=w3483:refnum<class "Channel.lvclass">, "Acquisition out"=w3495:refnum<class "Acquisition.lvclass">)  [unwired: 7 in]
              n1229 = call-dynamic "Write wait_expose.vi"("error in (no error)"=w3480, "wait_expose"=TRUE, "Channel in"=w3483) -> ("error out"=w3479:errorcluster, "Channel out"=w3482:refnum<class "Channel.lvclass">)  [unwired: 7 in]
              n1230 = call-dynamic "Read State Machine.vi"("error in (no error)"=w3479, "Device in"=w3482) -> ("error out"=w3490:errorcluster, "State Machine.lvclass"=w3492:refnum<class "State Machine.lvclass">, "Device out"=w3488:refnum<class "Channel.lvclass">)  [unwired: 7 in]
              n1231 = call "Next State.vi"("error in (no error)"=w3490, "New_State"=40, "State Machine in"=w3492) -> ("error out"=w3485:errorcluster, "State Machine out"=w3486:refnum<class "State Machine.lvclass">)  [unwired: 7 in]
              n1232 = call-dynamic "Write State Machine.vi"("error in (no error)"=w3485, "State Machine.lvclass"=w3486, "Device in"=w3488) -> ("error out"=w3487:errorcluster, "Device out"=w3489:refnum<class "Channel.lvclass">)  [unwired: 7 in]
              n1233 = call-dynamic "Write Channel.vi"("error in (no error)"=w3487, "Channel.lvclass"=w3489, "Acquisition in"=w3495) -> ("error out"=w3493:errorcluster, "Acquisition out"=w3494:refnum<class "Acquisition.lvclass">)  [unwired: 7 in]
            }
          }
          n1234 = call-dynamic "Write AcquisitionA.vi"("error in (no error)"=w3362, "Acquisition.lvclass"=w3364, "S4ACS_GUI in"=w3363) -> ("error out"=w3357:errorcluster, "S4ACS_GUI out"=w3358:refnum<class "S4GUI.lvclass">)  [unwired: 7 in]
          n1235 = call "Read AcquisitionB.vi"("error in (no error)"=w3357, "S4ACS_GUI in"=w3358) -> ("error out"=w3311:errorcluster, "Acquisition.lvclass"=w3313:refnum<class "Acquisition.lvclass">, "S4ACS_GUI out"=w3355:refnum<class "S4GUI.lvclass">)  [unwired: 7 in]
          n1236 = call-dynamic "Read enabled.vi"("error in (no error)"=w3311, "Server in"=w3313) -> ("error out"=w3310:errorcluster, "enabled"=w3300:bool, "Server out"=w3312:refnum<class "Acquisition.lvclass">)  [unwired: 7 in]
          n1237 = call "Read connection.vi"("error in (no error)"=w3310, "Server in"=w3312) -> ("error out"=w3338:errorcluster, "connection"=w3322:bool, "Server out"=w3339:refnum<class "Acquisition.lvclass">)  [unwired: 7 in]
          n1238 = And(x=w3322, y=w3300) -> (x .and. y?=w3323:bool)
          n1239 = case shown="True" w3323 {
            tunnel: w3339 -> [w3453 w3472]
            tunnel: w3338 -> [w3452 w3471]
            tunnel: [w3453 w3469] -> w3356
            tunnel: [w3452 w3468] -> w3354
            tunnel: [w3449 u32 0 ("New_State")] -> w3329
            tunnel: w3300 -> [w3448 _]
            frame False {
              n1240 = Select(t=u32 2, s=w3448, f=u32 0) -> (s? t:f=w3449:u32)
            }
            frame True {
              n1241 = call-dynamic "Read Channel.vi"("error in (no error)"=w3471, "Acquisition in"=w3472) -> ("error out"=w3455:errorcluster, "Channel.lvclass"=w3457:refnum<class "Channel.lvclass">, "Acquisition out"=w3470:refnum<class "Acquisition.lvclass">)  [unwired: 7 in]
              n1242 = call-dynamic "Write wait_expose.vi"("error in (no error)"=w3455, "wait_expose"=TRUE, "Channel in"=w3457) -> ("error out"=w3454:errorcluster, "Channel out"=w3456:refnum<class "Channel.lvclass">)  [unwired: 7 in]
              n1243 = call-dynamic "Read State Machine.vi"("error in (no error)"=w3454, "Device in"=w3456) -> ("error out"=w3465:errorcluster, "State Machine.lvclass"=w3467:refnum<class "State Machine.lvclass">, "Device out"=w3463:refnum<class "Channel.lvclass">)  [unwired: 7 in]
              n1244 = call "Next State.vi"("error in (no error)"=w3465, "New_State"=40, "State Machine in"=w3467) -> ("error out"=w3460:errorcluster, "State Machine out"=w3461:refnum<class "State Machine.lvclass">)  [unwired: 7 in]
              n1245 = call-dynamic "Write State Machine.vi"("error in (no error)"=w3460, "State Machine.lvclass"=w3461, "Device in"=w3463) -> ("error out"=w3462:errorcluster, "Device out"=w3464:refnum<class "Channel.lvclass">)  [unwired: 7 in]
              n1246 = call-dynamic "Write Channel.vi"("error in (no error)"=w3462, "Channel.lvclass"=w3464, "Acquisition in"=w3470) -> ("error out"=w3468:errorcluster, "Acquisition out"=w3469:refnum<class "Acquisition.lvclass">)  [unwired: 7 in]
            }
          }
          n1247 = call "Write AcquisitionB.vi"("error in (no error)"=w3354, "Acquisition.lvclass"=w3356, "S4ACS_GUI in"=w3355) -> ("error out"=w3350:errorcluster, "S4ACS_GUI out"=w3349:refnum<class "S4GUI.lvclass">)  [unwired: 7 in]
          n1248 = call-dynamic "Read AcquisitionC.vi"("error in (no error)"=w3350, "S4ACS_GUI in"=w3349) -> ("error out"=w3307:errorcluster, "Acquisition.lvclass"=w3309:refnum<class "Acquisition.lvclass">, "S4ACS_GUI out"=w3352:refnum<class "S4GUI.lvclass">)  [unwired: 7 in]
          n1249 = call-dynamic "Read enabled.vi"("error in (no error)"=w3307, "Server in"=w3309) -> ("error out"=w3306:errorcluster, "enabled"=w3299:bool, "Server out"=w3308:refnum<class "Acquisition.lvclass">)  [unwired: 7 in]
          n1250 = call "Read connection.vi"("error in (no error)"=w3306, "Server in"=w3308) -> ("error out"=w3336:errorcluster, "connection"=w3319:bool, "Server out"=w3337:refnum<class "Acquisition.lvclass">)  [unwired: 7 in]
          n1251 = And(x=w3319, y=w3299) -> (x .and. y?=w3321:bool)
          n1252 = case shown="True" w3321 {
            tunnel: [w3427 w3441] -> w3353
            tunnel: [w3428 w3440] -> w3351
            tunnel: w3337 -> [w3428 w3438]
            tunnel: w3336 -> [w3427 w3437]
            tunnel: [w3424 u32 0 ("New_State")] -> w3328
            tunnel: w3299 -> [w3423 _]
            frame False {
              n1253 = Select(t=u32 4, s=w3423, f=u32 0) -> (s? t:f=w3424:u32)
            }
            frame True {
              n1254 = call-dynamic "Read Channel.vi"("error in (no error)"=w3437, "Acquisition in"=w3438) -> ("error out"=w3430:errorcluster, "Channel.lvclass"=w3432:refnum<class "Channel.lvclass">, "Acquisition out"=w3439:refnum<class "Acquisition.lvclass">)  [unwired: 7 in]
              n1255 = call-dynamic "Write wait_expose.vi"("error in (no error)"=w3430, "wait_expose"=TRUE, "Channel in"=w3432) -> ("error out"=w3429:errorcluster, "Channel out"=w3431:refnum<class "Channel.lvclass">)  [unwired: 7 in]
              n1256 = call-dynamic "Read State Machine.vi"("error in (no error)"=w3429, "Device in"=w3431) -> ("error out"=w3444:errorcluster, "State Machine.lvclass"=w3442:refnum<class "State Machine.lvclass">, "Device out"=w3446:refnum<class "Channel.lvclass">)  [unwired: 7 in]
              n1257 = call "Next State.vi"("error in (no error)"=w3444, "New_State"=40, "State Machine in"=w3442) -> ("error out"=w3436:errorcluster, "State Machine out"=w3435:refnum<class "State Machine.lvclass">)  [unwired: 7 in]
              n1258 = call-dynamic "Write State Machine.vi"("error in (no error)"=w3436, "State Machine.lvclass"=w3435, "Device in"=w3446) -> ("error out"=w3447:errorcluster, "Device out"=w3445:refnum<class "Channel.lvclass">)  [unwired: 7 in]
              n1259 = call-dynamic "Write Channel.vi"("error in (no error)"=w3447, "Channel.lvclass"=w3445, "Acquisition in"=w3439) -> ("error out"=w3441:errorcluster, "Acquisition out"=w3440:refnum<class "Acquisition.lvclass">)  [unwired: 7 in]
            }
          }
          n1260 = call-dynamic "Write AcquisitionC.vi"("error in (no error)"=w3353, "Acquisition.lvclass"=w3351, "S4ACS_GUI in"=w3352) -> ("error out"=w3347:errorcluster, "S4ACS_GUI out"=w3346:refnum<class "S4GUI.lvclass">)  [unwired: 7 in]
          n1261 = call-dynamic "Read AcquisitionD.vi"("error in (no error)"=w3347, "S4ACS_GUI in"=w3346) -> ("error out"=w3303:errorcluster, "Acquisition.lvclass"=w3305:refnum<class "Acquisition.lvclass">, "S4ACS_GUI out"=w3345:refnum<class "S4GUI.lvclass">)  [unwired: 7 in]
          n1262 = call-dynamic "Read enabled.vi"("error in (no error)"=w3303, "Server in"=w3305) -> ("error out"=w3302:errorcluster, "enabled"=w3298:bool, "Server out"=w3304:refnum<class "Acquisition.lvclass">)  [unwired: 7 in]
          n1263 = call "Read connection.vi"("error in (no error)"=w3302, "Server in"=w3304) -> ("error out"=w3334:errorcluster, "connection"=w3318:bool, "Server out"=w3335:refnum<class "Acquisition.lvclass">)  [unwired: 7 in]
          n1264 = And(x=w3318, y=w3298) -> (x .and. y?=w3320:bool)
          n1265 = case shown="True" w3320 {
            tunnel: w3334 -> [w3402 w3422]
            tunnel: [w3402 w3421] -> w3348
            tunnel: w3335 -> [w3403 w3414]
            tunnel: [w3403 w3412] -> w3344
            tunnel: [w3399 u32 0 ("New_State")] -> w3327
            tunnel: w3298 -> [w3398 _]
            frame False {
              n1266 = Select(t=u32 8, s=w3398, f=u32 0) -> (s? t:f=w3399:u32)
            }
            frame True {
              n1267 = call-dynamic "Read Channel.vi"("error in (no error)"=w3422, "Acquisition in"=w3414) -> ("error out"=w3404:errorcluster, "Channel.lvclass"=w3407:refnum<class "Channel.lvclass">, "Acquisition out"=w3413:refnum<class "Acquisition.lvclass">)  [unwired: 7 in]
              n1268 = call-dynamic "Write wait_expose.vi"("error in (no error)"=w3404, "wait_expose"=TRUE, "Channel in"=w3407) -> ("error out"=w3405:errorcluster, "Channel out"=w3406:refnum<class "Channel.lvclass">)  [unwired: 7 in]
              n1269 = call-dynamic "Read State Machine.vi"("error in (no error)"=w3405, "Device in"=w3406) -> ("error out"=w3418:errorcluster, "State Machine.lvclass"=w3420:refnum<class "State Machine.lvclass">, "Device out"=w3416:refnum<class "Channel.lvclass">)  [unwired: 7 in]
              n1270 = call "Next State.vi"("error in (no error)"=w3418, "New_State"=40, "State Machine in"=w3420) -> ("error out"=w3410:errorcluster, "State Machine out"=w3411:refnum<class "State Machine.lvclass">)  [unwired: 7 in]
              n1271 = call-dynamic "Write State Machine.vi"("error in (no error)"=w3410, "State Machine.lvclass"=w3411, "Device in"=w3416) -> ("error out"=w3415:errorcluster, "Device out"=w3417:refnum<class "Channel.lvclass">)  [unwired: 7 in]
              n1272 = call-dynamic "Write Channel.vi"("error in (no error)"=w3415, "Channel.lvclass"=w3417, "Acquisition in"=w3413) -> ("error out"=w3421:errorcluster, "Acquisition out"=w3412:refnum<class "Acquisition.lvclass">)  [unwired: 7 in]
            }
          }
          n1273 = call-dynamic "Write AcquisitionD.vi"("error in (no error)"=w3348, "Acquisition.lvclass"=w3344, "S4ACS_GUI in"=w3345) -> ("error out"=w3343:errorcluster, "S4ACS_GUI out"=w3342:refnum<class "S4GUI.lvclass">)  [unwired: 7 in]
          n1274 = Compound Arithmetic op=ADD(w3330, w3329, w3328, w3327) -> (w3331:u32)
          n1275 = case shown="0, Default" w3331 {
            tunnel: w3326 -> [w3367 _ _ _ _ _ _ _ _ _ _ _ _ _ _ _]
            tunnel: [w3366 u32 1 ("Obs_state") u32 1 ("Obs_state") u32 1 ("Obs_state") u32 1 ("Obs_state") u32 1 ("Obs_state") u32 1 ("Obs_state") u32 1 ("Obs_state") u32 1 ("Obs_state") u32 1 ("Obs_state") u32 1 ("Obs_state") u32 1 ("Obs_state") u32 1 ("Obs_state") u32 1 ("Obs_state") u32 1 ("Obs_state") u32 1 ("Obs_state")] -> w3332
            tunnel: ["" ("Error Msg") "ERROR: Lost channel 1 connection... - HandleObservationSync.vi state 321" ("Error Msg") "ERROR: Lost channel 2 connection...- HandleObservationSync.vi state 321" ("Error Msg") "ERROR: Lost channels 1 and 2 connection...- HandleObservationSync.vi state 321" ("Error Msg") "ERROR: Lost channel 3 connection...- HandleObservationSync.vi state 321" ("Error Msg") "ERROR: Lost channels 1 and  3 connection...- HandleObservationSync.vi state 321" ("Error Msg") "ERROR:  Lost channels 2 and  3 connection...- HandleObservationSync.vi state 321" ("Error Msg") "ERROR:  Lost channels 1, 2 and  3 connection...- HandleObservationSync.vi state 321" ("Error Msg") "ERROR: Lost channel 4 connection...- HandleObservationSync.vi state 321" ("Error Msg") "ERROR:  Lost channels 1 and 4 connection...- HandleObservationSync.vi state 321" ("Error Msg") "ERROR:  Lost channels 2 and 4 connection...- HandleObservationSync.vi state 321" ("Error Msg") "ERROR: Lost channels 1, 2 and 4 connection...- HandleObservationSync.vi state 321" ("Error Msg") "ERROR: Lost channels 3 and 4 connection...- HandleObservationSync.vi state 321" ("Error Msg") "ERROR: Lost channels 1, 3 and 4 connection...- HandleObservationSync.vi state 321" ("Error Msg") "ERROR: Lost channels 2, 3 and 4 connection...- HandleObservationSync.vi state 321" ("Error Msg") "ERROR: Lost channels 1, 2, 3 and 4 connection...- HandleObservationSync.vi state 321" ("Error Msg")] -> w3333
            frame 0, Default {
              n1276 = Increment(x=w3367) -> (x+1=w3366:u32)
            }
            frame 1 {
            }
            frame 2 {
            }
            frame 3 {
            }
            frame 4 {
            }
            frame 5 {
            }
            frame 6 {
            }
            frame 7 {
            }
            frame 8 {
            }
            frame 9 {
            }
            frame 10 {
            }
            frame 11 {
            }
            frame 12 {
            }
            frame 13 {
            }
            frame 14 {
            }
            frame 15 {
            }
          }
          n1277 = Bundle By Name(cluster=w3342, "Obs_state"=w3332, "Error Msg"=w3333) -> (w3359:refnum<class "S4GUI.lvclass">)
        }
        frame 322 {
          # "Espera terminar o envio de WAIT EXPOSE COMMAND para todos os ACS."
